vi "Write Attribute Meta Data.vi"(6 "Meta Data":string, 7 "Linked List ID":string, 8 "error in (no error)":errorcluster, 9 "Attribute Type":variant, 10 "Attribute Name":string, 11 "Linked List in":refnum<class "Linked List.lvclass">) -> (0 "error out":errorcluster, 1 "Found?":bool, 3 "Linked List out":refnum<class "Linked List.lvclass">)   [LabVIEW 2019, in "Linked Lists.lvlib" / "Linked List.lvclass"]
uses:
  <vilib>/gpm_packages/@cs/linked-list/Source/Linked List/Linked List/Linked List.lvclass
  <vilib>/gpm_packages/@cs/linked-list/Source/Linked List/Linked List/Linked List.lvclass/Linked List.ctl
  <vilib>/gpm_packages/@cs/lookup-table/Source/LookupTable/LookupTable.lvclass/LookupTable.ctl
  6acb27cd-fb09-4806-a7e8-4cc67e1c4df2.vi
  b97af5a9-df1f-4a32-9975-07869ccef251.vi
  <vilib>/gpm_packages/@cs/lookup-table/Source/LookupTable/Read Table Reference.vi
  6acb27cd-fb09-4806-a7e8-4cc67e1c4df2.vi/ba17568b-cf65-4534-bc6d-97979592f511.vi
  b97af5a9-df1f-4a32-9975-07869ccef251.vi/5379ea23-07a5-4668-85fd-111a3777a90e.vi
  <vilib>/gpm_packages/@cs/lookup-table/Source/LookupTable/LookupTable.lvclass
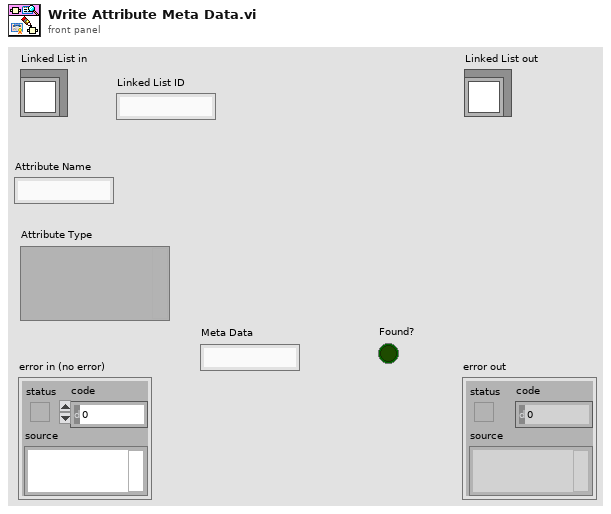
[diagram p1: front panel]
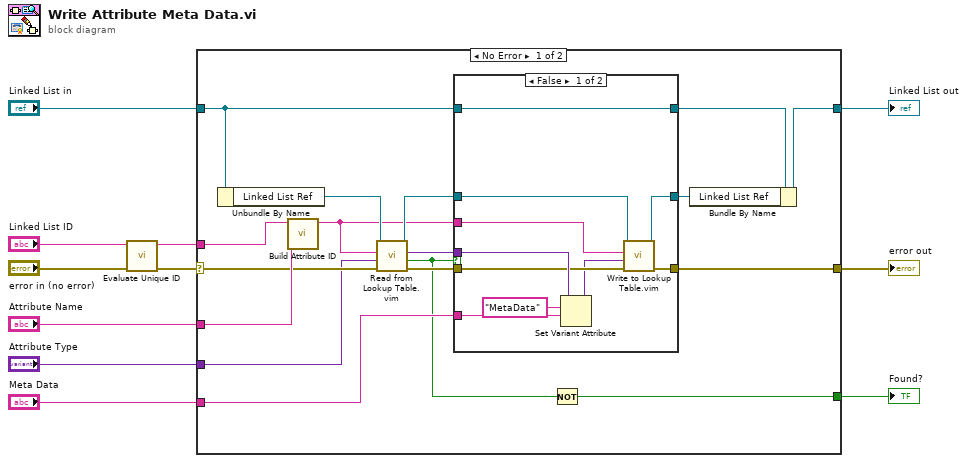
[diagram p0: block diagram]
diagram:
  n1 = call <vilib>:"Evaluate Unique ID.vi"("error in (no error)"="error in (no error)", "Unique ID"="Linked List ID") -> ("error out"=w11:errorcluster, "Unique ID Out"=w10:string)  [unwired: 8 in]
  n2 = case shown="No Error" w11 {
    selector: w11 -> [w25 w42]
    tunnel: w10 -> [w26 _]
    tunnel: "Linked List in" -> [w13 w43]
    tunnel: [w27 w43] -> w4
    tunnel: "Attribute Name" -> [w28 _]
    tunnel: "Attribute Type" -> [w23 _]
    tunnel: [w19 w42] -> w1
    tunnel: [w18 _] -> w2
    tunnel: "Meta Data" -> [w21 _]
    frame No Error {
      n3 = Unbundle By Name(w13) -> ("Linked List Ref"=w24:refnum<data-value>)
      n4 = call <vilib>:"Build Attribute ID.vi"("Attr Name"=w28, "Unique ID"=w26) -> ("Attr ID Out"=w15:string)  [unwired: 9 in]
      n5 = call "Read from Lookup Table.vim"("error in (no error)"=w25, "Type"=w23, "Item Name"=w15, "LookupTable Reference"=w24) -> ("error out"=w20:errorcluster, "Not Found?"=w14:bool, "Value"=w22:variant, "LookupTable Reference Out"=w17:refnum<data-value>)  [unwired: 4 in]
      n6 = case shown="False" w14 {
        tunnel: w22 -> [w38 _]
        tunnel: w21 -> [w36 _]
        tunnel: w20 -> [w35 w39]
        tunnel: [w34 w39] -> w19
        tunnel: w17 -> [w33 w40]
        tunnel: [w32 w40] -> w16
        tunnel: w15 -> [w31 _]
        tunnel: [w29 w41] -> w12
        tunnel: w13 -> [w29 w41]
        frame False {
          n7 = Set Variant Attribute(Variant=w38, name="MetaData", value=w36) -> (Variant out=w30:variant)  [unwired: 1 in, 2 out]
          n8 = call "Write to Lookup Table.vim"("error in (no error)"=w35, "Item"=w30, "Item Name"=w31, "LookupTable Reference"=w33) -> ("error out"=w34:errorcluster, "LookupTable Reference Out"=w32:refnum<data-value>)  [unwired: 5 in, 1 out]
        }
        frame True {
        }
      }
      n9 = Not(x=w14) -> (.not. x?=w18:bool)
      n10 = Bundle By Name(cluster=w12, "Linked List Ref"=w16) -> (w27:refnum<class "Linked List.lvclass">)
    }
    frame Error {
    }
  }
  "error out" <- w1
  "Linked List out" <- w4
  "Found?" <- w2
